vi "timekeeper clock servo.vi"   [LabVIEW 2011, in "EPS_Timekeeper.lvlib"]
uses:
  <vilib>/addons/Electrical Power/Example Support/PMU/Time Keeper/EPS_Timekeeper.lvlib
  <vilib>/addons/Electrical Power/Example Support/PMU/Time Keeper/timekeeper clock servo state.ctl
  <vilib>/rvi/FXPMathLib/FxpDiv/subVIs/nifxpmath_Div_SimConfig.ctl
  <vilib>/addons/Electrical Power/Example Support/PMU/Time Keeper/timekeeper timereference time (g).vi
  <vilib>/addons/Electrical Power/Example Support/PMU/Time Keeper/timekeeper timereference timestamp (g).vi
  <vilib>/addons/Electrical Power/Example Support/PMU/Time Keeper/timekeeper locked (g).vi
  <vilib>/addons/Electrical Power/Example Support/PMU/Time Keeper/timekeeper offset from timeref (g).vi
  <vilib>/rvi/FXPMathLib/FxpDiv/simVIs/DllFxpDivTemp_sub.vi
  <vilib>/rvi/FXPMathLib/FxpMul/XNode/nifxpmath_Multiplier.xnode
  <vilib>/rvi/FXPMathLib/FxpDiv/XNode/nifxpmath_Div.xnode
  <vilib>/rvi/FXPMathLib/sim/FxpSim.dll
types:
  T1 = typedef "EPS_Timekeeper.lvlib/timekeeper clock servo state.ctl" = enum8{"AdjustTime", "AdjustFrequency", "AdjustPhase"}
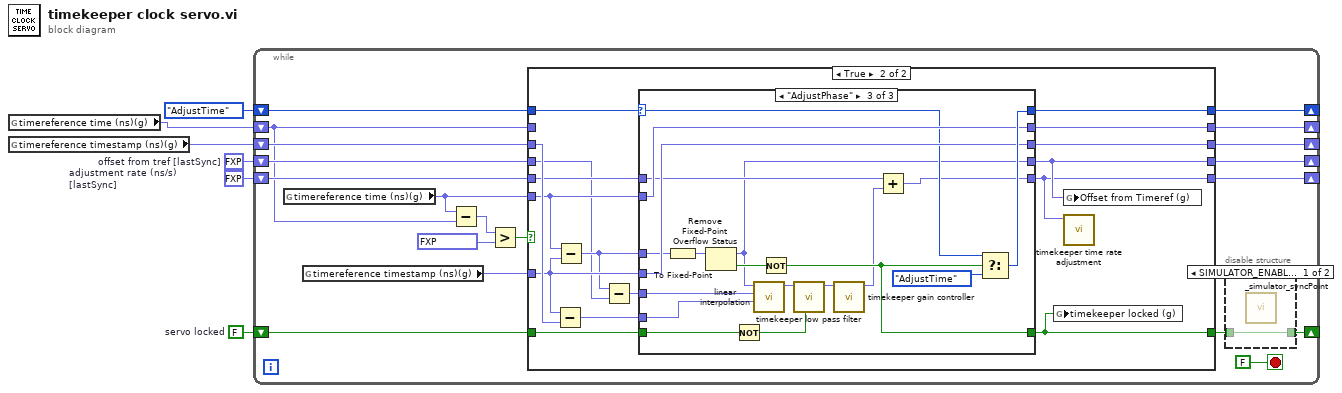
[diagram p0: block diagram]
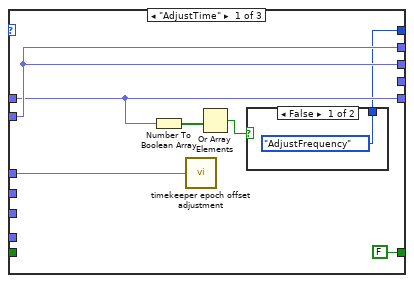
[diagram p4: hidden frame]
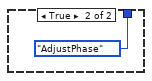
[diagram p5: hidden frame]
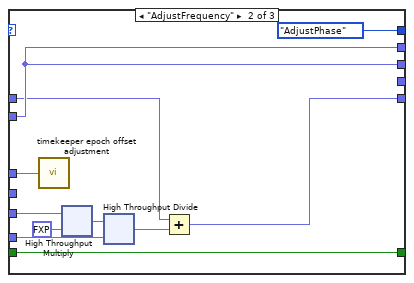
[diagram p6: hidden frame]
diagram:
  w3 = FALSE  # servo locked
  w4 = fxp<+/-,19,19> 0.0  # adjustment rate (ns/s) [lastSync]
  w5 = fxp<+/-,21,21> 0.0  # offset from tref [lastSync]
  n1 = global read "timekeeper timereference time (g).vi" "timereference time (ns)(g)"() -> (w1:fxp<+,64,64>)
  n2 = global read "timekeeper timereference timestamp (g).vi" "timereference timestamp (ns)(g)"() -> (w2:fxp<+,64,64>)
  n3 = while {
    shift-right: [w20] -> _
    shift-left: timekeeper_clock_servo_state."AdjustTime" ("timekeeper clock servo state") -> [w12]
    shift-right: [w23] -> _
    shift-left: w1 -> [w10]
    shift-right: [w22] -> _
    shift-left: w2 -> [w11]
    shift-right: [w21] -> _
    shift-left: w5 -> [w24]
    shift-right: [w8] -> _
    shift-left: w4 -> [w19]
    shift-right: [w15] -> _
    shift-left: w3 -> [w18]
    stop <- FALSE stop-if-true
    n4 = global read "timekeeper timereference time (g).vi" "timereference time (ns)(g)"() -> (w9:fxp<+,64,64>)
    n5 = global read "timekeeper timereference timestamp (g).vi" "timereference timestamp (ns)(g)"() -> (w7:fxp<+,64,64>)
    n6 = Subtract(x=w9, y=w10) -> (x-y=w14:fxp<+,30,30>)
    n7 = Greater?(x=w14, y=fxp<+,23,30> 950000000.0) -> (0:w13:bool)
    n8 = case shown="True" w13 {
      tunnel: w9 -> [_ w39]
      tunnel: w7 -> [_ w40]
      tunnel: w12 -> [w33 w42]
      tunnel: w11 -> [w31 w46]
      tunnel: w24 -> [w30 w36]
      tunnel: w10 -> [w32 _]
      tunnel: [w32 w49] -> w23
      tunnel: [w31 w48] -> w22
      tunnel: [w30 w43] -> w21
      tunnel: [w33 w35] -> w20
      tunnel: w19 -> [w29 w38]
      tunnel: [w29 w34] -> w8
      tunnel: w18 -> [w28 w45]
      tunnel: [w28 w44] -> w16
      frame False {
      }
      frame True {
        n9 = Subtract(x=w40, y=w46) -> (x-y=w47:fxp<+/-,32,32>)
        n10 = Subtract(x=w39, y=w40) -> (x-y=w37:fxp<+/-,64,64>)
        n11 = Subtract(x=w37, y=w36) -> (x-y=w41:fxp<+/-,18,18>)
        n12 = case shown="\"AdjustPhase\"" w42 {
          selector: w42 -> [_ _ w111]
          tunnel: w37 -> [w55 w68 w106]
          tunnel: w40 -> [_ _ w112]
          tunnel: w39 -> [w56 w65 w113]
          tunnel: [w56 w65 w113] -> w49
          tunnel: [w56 w65 w112] -> w48
          tunnel: [_ _ w99] -> w43
          tunnel: [w50 timekeeper_clock_servo_state."AdjustPhase" ("timekeeper clock servo state") w114] -> w35
          tunnel: w47 -> [_ w59 w97]
          tunnel: w41 -> [_ w63 w98]
          tunnel: [w52 w61 w100] -> w34
          tunnel: w45 -> [_ w66 w110]
          tunnel: [FALSE ("servo locked") w66 w103] -> w44
          tunnel: w38 -> [w52 w62 w102]
          frame "AdjustTime" {
            n13 = Number To Boolean Array(number=w52) -> (Boolean array=w53:bool[])
            n14 = call <vilib>:"timekeeper epoch offset adjustment.vi"("offset"=w55) -> ()
            n15 = Or Array Elements(Boolean array=w53) -> (logical OR=w51:bool)
            n16 = case shown="False" w51 {
              tunnel: [timekeeper_clock_servo_state."AdjustFrequency" ("timekeeper clock servo state") timekeeper_clock_servo_state."AdjustPhase" ("timekeeper clock servo state")] -> w50
              frame False {
              }
              frame True {
              }
            }
          }
          frame "AdjustFrequency" {
            n17 = call <vilib>:"timekeeper epoch offset adjustment.vi"("offset"=w68) -> ()
            n18 = xnode "High Throughput Multiply"("x"=w63, "y"=fxp<+,30,30> 1000000000.0) -> ("x*y"=w60:fxp<+/-,48,48>)
            n19 = xnode "High Throughput Divide"("x"=w60, "y"=w59) -> ("x/y"=w67:fxp<+/-,18,18>)
            n20 = Add(x=w62, y=w67) -> (x+y=w61:fxp<+/-,19,19>)
          }
          frame "AdjustPhase" {
            n21 = To Fixed-Point(number=w106) -> (fixed-point=w104:fxp<+/-,19,19>)  [unwired: 1 in]
            n22 = Remove Fixed-Point Overflow Status(3:w104) -> (0:w105:bool, 1:w99:fxp<+/-,19,19>)
            n23 = Not(x=w110) -> (.not. x?=w109:bool)
            n24 = call <vilib>:"linear interpolation.vi"("dx"=w97, "dy"=w98, "y"=w99) -> ("predicted y"=w108:fxp<+/-,24,24>)  [unwired: 4 in]
            n25 = Not(x=w105) -> (.not. x?=w103:bool)
            n26 = call <vilib>:"timekeeper low pass filter.vi"("Initialize"=w109, "offset"=w108) -> ("filtered offset"=w107:fxp<+/-,24,24>)  [unwired: 6 in]
            n27 = call <vilib>:"timekeeper gain controller.vi"("offset"=w107) -> ("adjustment rate (ns/s)"=w101:fxp<+/-,21,21>)  [unwired: 7 in]
            n28 = Add(x=w102, y=w101) -> (x+y=w100:fxp<+/-,19,19>)
            n29 = Select(t=w111, s=w103, f=timekeeper_clock_servo_state."AdjustTime" ("timekeeper clock servo state")) -> (s? t:f=w114:T1)
          }
        }
        n30 = global write "timekeeper locked (g).vi" "timekeeper locked (g)"(w44) -> ()
        n31 = global write "timekeeper offset from timeref (g).vi" "Offset from Timeref (g)"(w43) -> ()
        n32 = call <vilib>:"timekeeper time rate adjustment.vi"("offset"=w34) -> ()  [unwired: 7 in]
      }
    }
    n33 = disable-structure shown="SIMULATOR_ENABLED==TRUE" {
      disable-tunnel: w16 -> [w26 w27]
      disable-tunnel: [w26 w27] -> w15
      frame condition #0 {
        n34 = call <vilib>:"_simulator_syncPoint.vi"() -> ()  [unwired: 12 in]
      }
      frame condition #1 (active) {
      }
    }
  }
